vi "IndexControl.vi"(8 "Power":dbl, 9 "Chamber":bool, 10 "Back":bool, 11 "Forward":bool) -> (2 "Numeric":dbl)   [LabVIEW 2011]
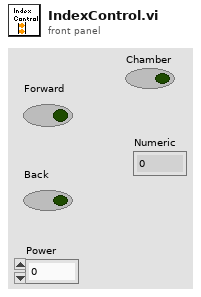
[diagram p1: front panel]
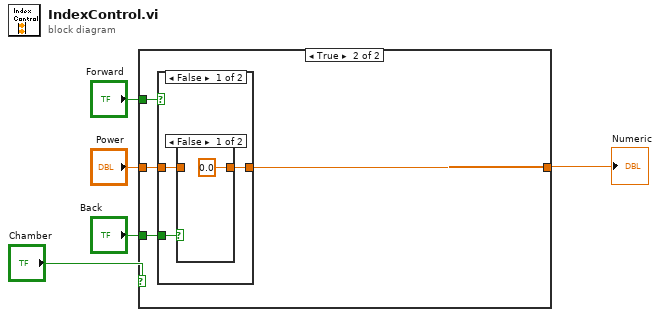
[diagram p0: block diagram]
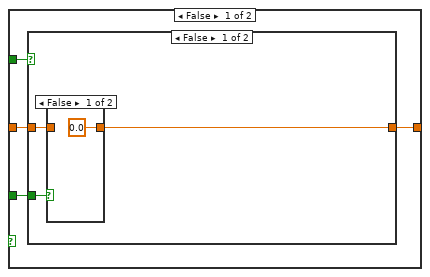
[diagram p2: hidden frame]
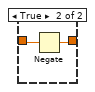
[diagram p3: hidden frame]
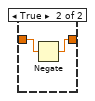
[diagram p5: hidden frame]
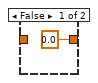
[diagram p7: hidden frame]
diagram:
  n1 = case shown="True" "Chamber" {
    tunnel: "Forward" -> [w9 w18]
    tunnel: "Power" -> [w8 w19]
    tunnel: [w7 w20] -> w3
    tunnel: "Back" -> [w6 w17]
    frame False {
      n2 = case shown="False" w9 {
        tunnel: w8 -> [w11 w16]
        tunnel: [w10 w16] -> w7
        tunnel: w6 -> [w12 _]
        frame False {
          n3 = case shown="False" w12 {
            tunnel: w11 -> [_ w14]
            tunnel: [0.0 w15] -> w10
            frame False {
            }
            frame True {
              n4 = Negate(x=w14) -> (-x=w15:dbl)
            }
          }
        }
        frame True {
        }
      }
    }
    frame True {
      n5 = case shown="False" w18 {
        tunnel: w19 -> [w23 w27]
        tunnel: [w22 w29] -> w20
        tunnel: w17 -> [w21 w28]
        frame False {
          n6 = case shown="False" w21 {
            tunnel: w23 -> [_ w25]
            tunnel: [0.0 w26] -> w22
            frame False {
            }
            frame True {
              n7 = Negate(x=w25) -> (-x=w26:dbl)
            }
          }
        }
        frame True {
          n8 = case shown="True" w28 {
            tunnel: [0.0 w31] -> w29
            tunnel: w27 -> [_ w31]
            frame False {
            }
            frame True {
            }
          }
        }
      }
    }
  }
  "Numeric" <- w3
